vi "Open Explore States Dialog.vi"(8 "error in (no error)":errorcluster, 11 "Owning VI Details":T1) -> (0 "error out":errorcluster)   [LabVIEW 2020]
uses:
  synchronization/synchronization.lvclass
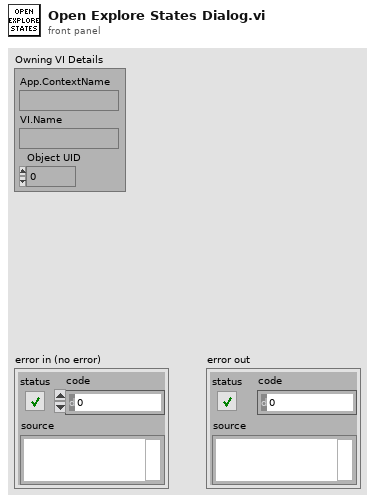
[diagram p1: front panel]
types:
  T1 = cluster{"App.ContextName":string, "VI.Name":string, "Object UID":i32}
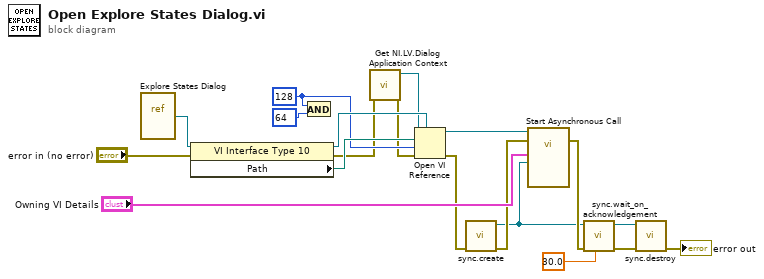
[diagram p0: block diagram]
diagram:
  w13 = 128 ("options")
  n1 = vi-ref "Explore States Dialog.vi"() -> (w19:refnum<vi>)
  n2 = property class="VI Interface Type 10"(reference=w19, error in="error in (no error)") -> (reference out=w15:refnum<vi>, error out=w11:errorcluster, "Path"=w18:path)
  n3 = And(x=w13, y=64 ("options")) -> ()  [unwired: 1 out]
  n4 = call "Get NI.LV.Dialog Application Context.vi"("error in (no error)"=w11) -> ("error out"=w10:errorcluster, "Application out"=w12:refnum<vi>)  [unwired: 9 in]
  n5 = Open VI Reference(type specifier VI Refnum (for type only)=w15, application reference (local)=w12, vi path=w18, options=w13, error in (no error)=w10) -> (vi reference=w16:refnum<vi>, error out=w6:errorcluster)  [unwired: 1 out]
  n6 = call "sync.create.vi"("error in (no error)"=w6) -> ("error out"=w5:errorcluster, "synchronization"=w1:refnum<class "synchronization.lvclass">)  [unwired: 9 in]
  n7 = call-by-ref "Start Asynchronous Call"(reference=w16, error in=w5, "synchronization"=w1, "Owning VI Details"="Owning VI Details") -> (error out=w4:errorcluster)  [unwired: 9 in, 2 out]
  n8 = call "sync.wait_on_acknowledgement.vi"("timeout (30s)"=30.0 ("timeout (10s)"), "error in (no error)"=w4, "synchronization in"=w1) -> ("error out"=w8:errorcluster, "synchronization out"=w2:refnum<class "synchronization.lvclass">)  [unwired: 7 in]
  n9 = call "sync.destroy.vi"("error in (no error)"=w8, "synchronization"=w2) -> ("error out"=→"error out":errorcluster)  [unwired: 9 in]
